vi "SigGen_NIRF_MatchIDNStr.vi"(8 "error in":errorcluster, 10 "IDNStr":string) -> (0 "error out":errorcluster, 2 "IDN match":bool, 3 "ClassLibraryFile":path)   [LabVIEW 2014]
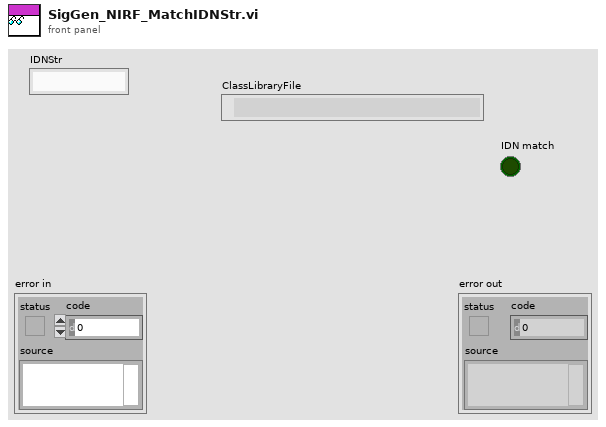
[diagram p1: front panel]
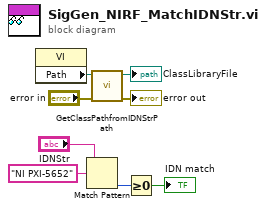
[diagram p0: block diagram]
diagram:
  n1 = property class="VI"() -> ("Path"=w8:path)  [unwired: 2 in, 2 out]
  n2 = Match Pattern(string="IDNStr", regular expression="NI PXI-5652") -> (offset past match=w2:i32)  [unwired: 1 in, 3 out]
  n3 = call "GetClassPathfromIDNStrPath.vi"("error in (no error)"="error in", "Path in"=w8) -> ("error out"=→"error out":errorcluster, "Path out"=→"ClassLibraryFile":path)  [unwired: 8 in]
  n4 = Greater Or Equal To 0?(x=w2) -> (x >= 0?=→"IDN match":bool)
